vi "ControlTable.vi"(0 "Data In":T4, 2 "Display State In":T2 items=["not ready", "ready"], 3 "Container State":T3) -> (6 "Data Out":T4, 7 "Display State Out":T2 items=["not ready", "ready"], 8 "Action":T1)   [LabVIEW 2018, in "XControl _Table.xctl"]
uses:
  XControl _Table.xctl
  TableData.ctl
  <vilib>/_xctls/Container State.ctl
  TableState.ctl
  <vilib>/_xctls/Action.ctl
  <vilib>/_xctls/XControlSupport.lvlib
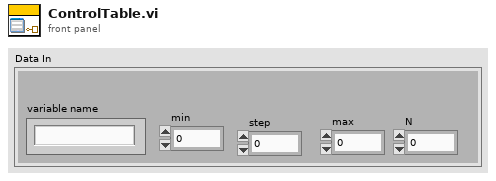
[diagram p1: front panel]
types:
  T1 = typedef "XControlSupport.lvlib/Action.ctl" = cluster{"Data Changed?":bool, "State Changed?":bool, "Action Name":string}
  T2 = typedef "XControl _Table.xctl/TableState.ctl" = u16
  T3 = typedef "XControlSupport.lvlib/Container State.ctl" = cluster{"Indicator?":bool, "Run Mode?":bool, " Refnum":refnum<vi>}
  T4 = typedef "XControl _Table.xctl/TableData.ctl" = cluster{"variable name":string, "min":dbl, "step":dbl, "max":dbl, "N":dbl}
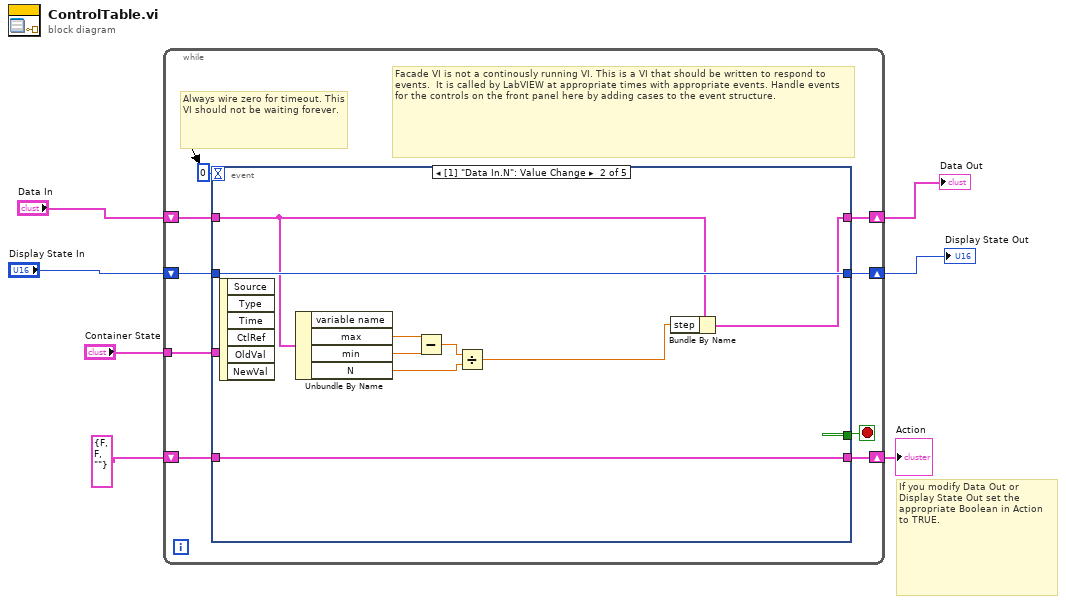
[diagram p0: block diagram]
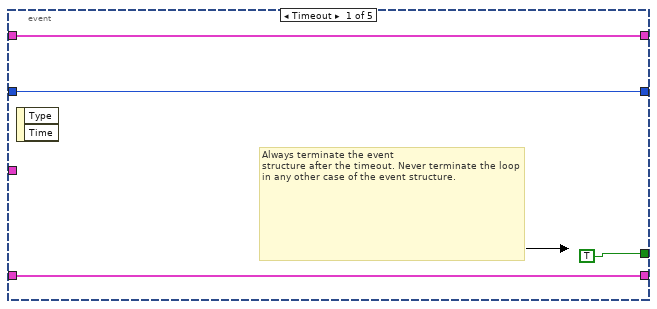
[diagram p2: hidden frame]
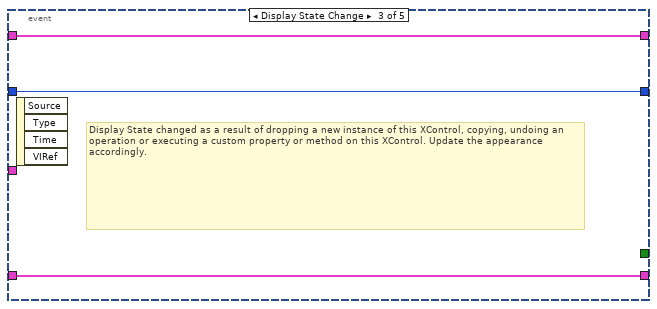
[diagram p3: hidden frame]
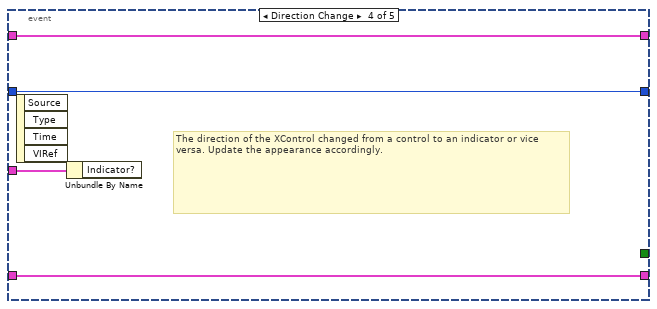
[diagram p4: hidden frame]
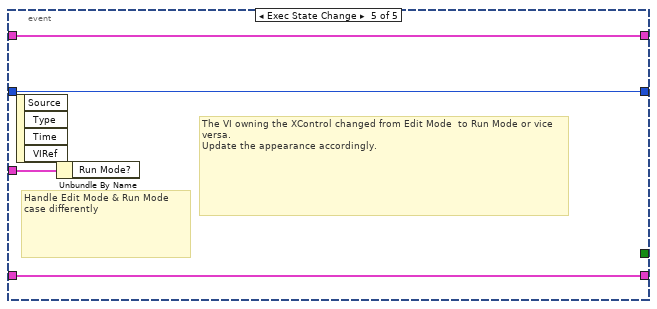
[diagram p5: hidden frame]
diagram:
  # "If you modify Data Out or\nDisplay State Out set the\nappropriate Boolean in Action\nto TRUE."
  n1 = while {
    shift-right: [w15] -> w4
    shift-left: "Display State In" -> [w16]
    tunnel: "Container State" -> [w12]
    shift-right: [w10] -> w7
    shift-left: "Data In" -> [w11]
    shift-right: [w8] -> w2
    shift-left: T1 {"Data Changed?"=FALSE, "State Changed?"=FALSE, "Action Name"=""} ("Action") -> [w9]
    stop <- w14 stop-if-true
    # "Facade VI is not a continously running VI. This is a VI that should be written to respond to events.  It is called by LabVIEW at appropriate times with appropriate events. Handle events for the controls on the front panel here by adding cases to the event structure."
    # "Always wire zero for timeout. This\nVI should not be waiting forever."
    n2 = event shown="[1] \"Data In.N\": Value Change" {
      selector: _ -> [_ _ _ _ _]
      dyn-events: _ -> [_ _ _ _ _]
      timeout: 0 -> [_ _ _ _ _]
      tunnel: w16 -> [w18 w29 w32 w35 w39]
      tunnel: [w18 w29 w32 w35 w39] -> w15
      tunnel: [TRUE _ _ _ _] -> w14
      tunnel: w12 -> [_ _ _ w36 w40]
      tunnel: w11 -> [w17 w27 w31 w34 w38]
      tunnel: [w17 w26 w31 w34 w38] -> w10
      tunnel: [w19 w28 w30 w33 w37] -> w8
      tunnel: w9 -> [w19 w28 w30 w33 w37]
      event Timeout {
        # "Always terminate the event\nstructure after the timeout. Never terminate the loop in any other case of the event structure."
        n3 = event-data() -> ()  [unwired: 1 in, 2 out]
      }
      event Value Change {
        n4 = event-data() -> ()  [unwired: 1 in, 6 out]
        n5 = Unbundle By Name(w27) -> ("max"=w25:dbl, "min"=w24:dbl, "N"=w22:dbl)  [unwired: 1 out]
        n6 = Subtract(x=w25, y=w24) -> (x-y=w23:dbl)
        n7 = Divide(x=w23, y=w22) -> (x/y=w21:dbl)
        n8 = Bundle By Name(cluster=w27, "step"=w21) -> (w26:T4)
      }
      event Display State Change {
        # "Display State changed as a result of dropping a new instance of this XControl, copying, undoing an operation or executing a custom property or method on this XControl. Update the appearance accordingly."
        n9 = event-data() -> ()  [unwired: 1 in, 4 out]
      }
      event Direction Change {
        # "The direction of the XControl changed from a control to an indicator or vice versa. Update the appearance accordingly."
        n10 = event-data() -> ()  [unwired: 1 in, 4 out]
        n11 = Unbundle By Name(w36) -> ()  [unwired: 1 out]
      }
      event Exec State Change {
        # "The VI owning the XControl changed from Edit Mode  to Run Mode or vice versa.\nUpdate the appearance accordingly."
        # "Handle Edit Mode & Run Mode\ncase differently"
        n12 = event-data() -> ()  [unwired: 1 in, 4 out]
        n13 = Unbundle By Name(w40) -> ()  [unwired: 1 out]
      }
    }
  }
  "Display State Out" <- w4
  "Data Out" <- w7
  "Action" <- w2
